vi "USB cmd send, wait for ACK.vi"(4 "Wait for ACK?":bool, 6 "Error In":errorcluster, 7 "4 byte config str":string, 8 "Cmd":T1="P", 9 "VISA resource name in":refnum<visa-resource-name>) -> (0 "Error out":errorcluster, 1 "Return msg":string, 2 "ACK ok":bool, 3 "VISA resource name out":refnum<visa-resource-name>)   [LabVIEW 2015]
uses:
  Ctls/Cmd str.ctl
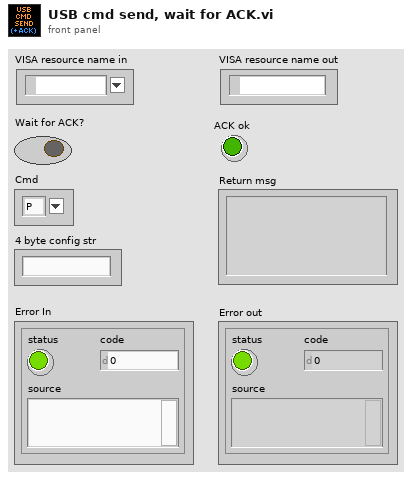
[diagram p1: front panel]
types:
  T1 = typedef "Cmd str.ctl" = string
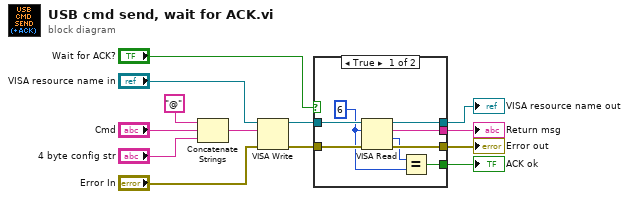
[diagram p0: block diagram]
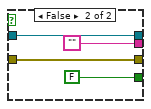
[diagram p2: hidden frame]
diagram:
  n1 = Concatenate Strings("@" ("string"), "Cmd", "4 byte config str") -> (w2:string)
  n2 = VISA Write(VISA resource name="VISA resource name in", write buffer=w2, error in (no error)="Error In") -> (VISA resource name out=w9:refnum<visa-resource-name>, error out=w7:errorcluster)  [unwired: 1 out]
  n3 = case shown="True" "Wait for ACK?" {
    tunnel: w9 -> [w21 w25]
    tunnel: [w20 w25] -> w8
    tunnel: w7 -> [w19 w24]
    tunnel: [w18 w24] -> w6
    tunnel: [w17 "" ("read buffer")] -> w5
    tunnel: [w14 FALSE] -> w4
    frame True {
      w15 = u32 6 ("byte count")
      n4 = VISA Read(VISA resource name=w21, byte count=w15, error in (no error)=w19) -> (VISA resource name out=w20:refnum<visa-resource-name>, read buffer=w17:string, return count=w16:u32, error out=w18:errorcluster)
      n5 = Equal?(x=w16, y=w15) -> (x = y?=w14:bool)
    }
    frame False {
    }
  }
  "Error out" <- w6
  "VISA resource name out" <- w8
  "Return msg" <- w5
  "ACK ok" <- w4
